vi "Ch Set Comm State.vi"(9 "pstRsdcb":T1, 10 "Channel":u8, 11 "devId":i32) -> (1 "pstRsdcb out":T1, 2 "devId out":i32, 3 "function return":i32)   [LabVIEW 2013, in "CHR34XXX.lvlib"]
doc: "DLL BOOL __stdcall CHR34XXX_Ch_SetCommState(IN int devId,IN BYTE Channel,IN pCHRUART_DCB_ST pstRsdcb);"
uses:
  CHR34XXX.lvlib
  CHR34XXX.dll
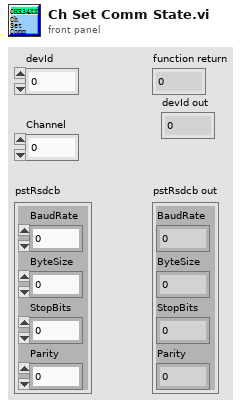
[diagram p1: front panel]
types:
  T1 = cluster{"BaudRate":u32, "ByteSize":u32, "StopBits":u32, "Parity":u32}
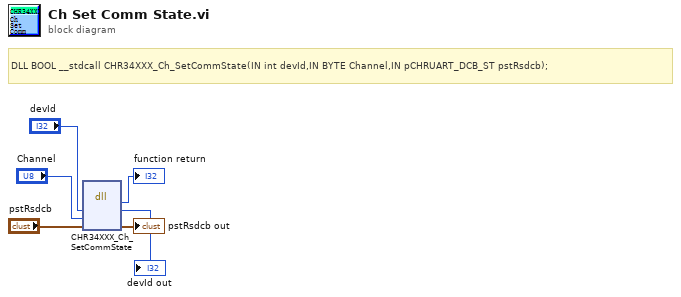
[diagram p0: block diagram]
diagram:
  # "DLL BOOL __stdcall CHR34XXX_Ch_SetCommState(IN int devId,IN BYTE Channel,IN pCHRUART_DCB_ST pstRsdcb);"
  n1 = dll-call lib="C:/Users/dy/Desktop/CHR34XXX_lv/lv_lib/CHR34XXX.*" fn="CHR34XXX_Ch_SetCommState"("devId"="devId", "Channel"="Channel", "pstRsdcb"="pstRsdcb") -> ("返回类型"=→"function return":i32, "devId"=→"devId out":i32, "pstRsdcb"=→"pstRsdcb out":T1)  [unwired: 4 in, 2 out]
